vi "Initialise Routes.vi"(8 "error in (no error)":errorcluster, 11 "Main Overlay":refnum<k24>) -> (0 "error out":errorcluster)   [LabVIEW 2014]
uses:
  C:/Robotic Systems/Products/Surveyor/Software/Ground Station/Data/Mapping DLL/GMap.NET.WindowsForms.dll
  Data/Mapping DLL/GMap.NET.WindowsForms.dll
  System.Drawing
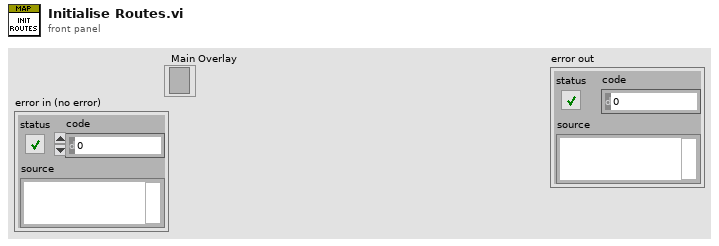
[diagram p1: front panel]
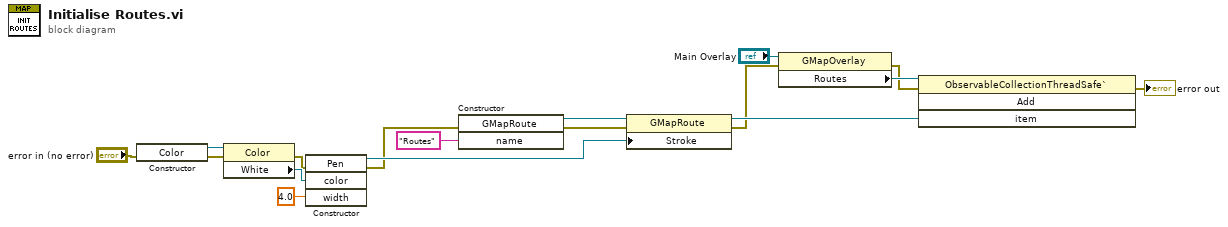
[diagram p0: block diagram]
diagram:
  n1 = constructor class="Color"(error in="error in (no error)") -> (reference out=w14:refnum<k24>, error out=w9:errorcluster)  [unwired: 2 in, 1 out]
  n2 = property class="Color"(reference=w14, error in=w9) -> (error out=w8:errorcluster, "White"=w12:refnum<k24>)  [unwired: 1 out]
  n3 = constructor class="Pen"(error in=w8, "color"=w12, "width"=sgl 4.0 ("Width")) -> (reference out=w13:refnum<k24>, error out=w7:errorcluster)  [unwired: 2 in, 3 out]
  n4 = constructor class="GMapRoute"(error in=w7, "name"="Routes") -> (reference out=w16:refnum<k24>, error out=w15:errorcluster)  [unwired: 2 in, 2 out]
  n5 = property class="GMapRoute"(reference=w16, error in=w15, "Stroke"=w13) -> (reference out=w11:refnum<k24>, error out=w3:errorcluster)
  n6 = property class="GMapOverlay"(reference="Main Overlay", error in=w3) -> (error out=w2:errorcluster, "Routes"=w4:refnum<k24>)  [unwired: 1 out]
  n7 = invoke class="ObservableCollectionThreadSafe`" method="Add"(reference=w4, error in=w2, "item"=w11) -> (error out=→"error out":errorcluster)  [unwired: 1 in, 3 out]
